vi "ma_SML Exponential Weighting.vi"   [LabVIEW 2020, in "NI_MAPro.lvlib"]
uses:
  NI_MAPro.lvlib
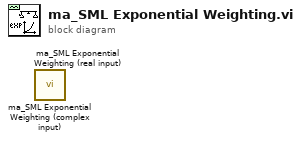
[diagram p0: block diagram]
diagram:
  n1 = call "ma_SML Exponential Weighting (complex input).vi"() -> ()  [unwired: 3 in, 2 out]
  n2 = call "ma_SML Exponential Weighting (real input).vi"() -> ()  [unwired: 3 in, 2 out]
